vi "Useless Machine singlethread test.vi"   [LabVIEW 2014]
uses:
  <vilib>/NXT/Block Support/NXT_InputPort.ctl
  <vilib>/NXT/Block Support/NXT_OutputPort.ctl
  <vilib>/NXT/Dual Mode Library/Sound/Tone.vi
  <vilib>/NXT/Dual Mode Library/Waits/Wait_LetGo.vi
  <vilib>/NXT/NXTIO Xnodes/NXTIONodeSubVIs/NXTMoveMotors.vi
  <vilib>/NXT/Dual Mode Library/Waits/Wait_Touch.vi
  <vilib>/NXT/NXTIO Xnodes/NXTIONodeSubVIs/NXTStopMotors.vi
  <vilib>/NXT/NXTIO Xnodes/AddressXNode/NXTIOAddress.xnode
  <vilib>/NXT/NXTIO Xnodes/NXTIOXNode/NXTIO.xnode
  <vilib>/NXT/Subs/LVHSConnector.ctl
  <vilib>/NXT/LegoClasses/BrickReference/BrickReference.lvclass
types:
  T1 = typedef "NXT_InputPort.ctl" = u32
  T2 = typedef "LVHSConnector.ctl" = refnum<class "BrickReference.lvclass">
  T3 = typedef "NXT_OutputPort.ctl" = u8
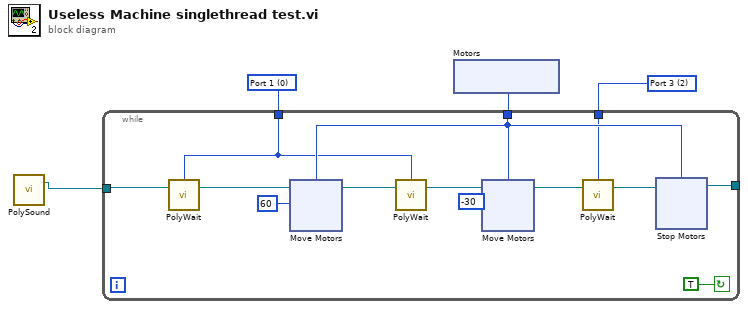
[diagram p0: block diagram]
diagram:
  w1 = T1 2 items=["Port 1", "Port 2", "Port 3", "Port 4"] ("Port (Port 1)")
  w2 = T1 0 items=["Port 1", "Port 2", "Port 3", "Port 4"] ("Port (Port 1)")
  n1 = call-poly <vilib>:"PolySound.vi"() -> ("NXT/EV3"=w3:T2)  [unwired: 4 in]
  n2 = xnode "Motors"() -> ("Motor"=w4:T3)
  n3 = while {
    tunnel: w4 -> [w13]
    tunnel: w3 -> [w8]
    tunnel: w2 -> [w10]
    tunnel: w1 -> [w6]
    tunnel: [w5] -> _
    stop <- TRUE continue-if-true
    n4 = call-poly <vilib>:"PolyWait.vi"("NXT/EV3"=w8, "Port (Port 1)"=w10) -> ("NXTEV3"=w11:T2)  [unwired: 2 in]
    n5 = xnode "Move Motors"("Power/Speed 1"=i8 60, "Motors"=w13, "NXT/EV3"=w11) -> ("NXT/EV3"=w12:T2)
    n6 = call-poly <vilib>:"PolyWait.vi"("NXT/EV3"=w12, "Port (Port 1)"=w10) -> ("NXT/EV3"=w9:T2)  [unwired: 2 in]
    n7 = xnode "Move Motors"("Power/Speed 1"=i8 -30, "Motors"=w13, "NXT/EV3"=w9) -> ("NXT/EV3"=w17:T2)
    n8 = call-poly <vilib>:"PolyWait.vi"("NXT/EV3"=w17, "Port (Port 1)"=w6) -> ("NXT/EV3"=w16:T2)  [unwired: 2 in]
    n9 = xnode "Stop Motors"("Motors"=w13, "NXT/EV3"=w16) -> ("NXT/EV3"=w5:T2)
  }
